vi "CheckIDchange.vi"(11 "ID":i32) -> (3 "ID change":bool)   [LabVIEW 2017]
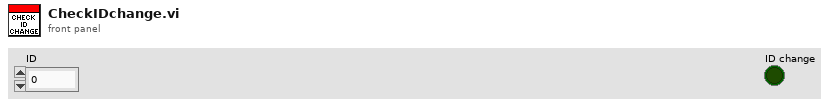
[diagram p1: front panel]
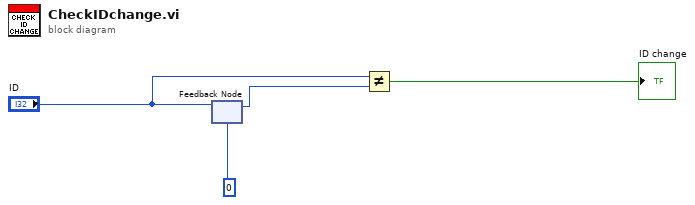
[diagram p0: block diagram]
diagram:
  n1 = feedback-in #1("ID") -> ()
  n2 = feedback #1(0 ("ID")) -> (w3:i32)
  n3 = Not Equal?(x="ID", y=w3) -> (x != y?=→"ID change":bool)
